vi "(SubVI)_2Ddisplay_direct_doppler_Ver6.vi"(0 "Data":dbl[][](array[numeric]), 1 "Image Avg 2D":dbl, 5 "zero array":dbl[][](array[numeric])=array250x513[128250 elements], 7 "first row":dbl[](array[numeric])=[0.0, 0.69647, 1.3934, 2.0908, 2.7886, 3.4868, 4.1855, 4.8847, 5.5842, 6.2843, 6.9848, 7.6857, 8.3871, 9.0889, 9.7912, 10.494, 11.197, 11.901, 12.605, 13.309, 14.014, 14.72, 15.426, 16.132, 16.839, 17.546, 18.254, 18.962, 19.67, 20.379, 21.089, 21.799, 22.509, 23.22, 23.932, 24.643, 25.356, 26.068, 26.781, 27.495, 28.209, 28.924, 29.639, 30.354, 31.07, 31.786, 32.503, 33.221, 33.938, 34.656, 35.375, 36.094, 36.814, 37.534, 38.255, 38.976, 39.697, 40.419, 41.141, 41.864, 42.588, 43.311, 44.036, 44.76, 45.486, 46.211, 46.937, 47.664, 48.391, 49.119, 49.847, 50.575, 51.304, 52.034, 52.763, 53.494, 54.225, 54.956, 55.688, 56.42, 57.153, 57.886, 58.62, 59.354, 60.089, 60.824, 61.559, 62.295, 63.032, 63.769, 64.506, 65.244, 65.983, 66.722, 67.461, 68.201, 68.942, 69.683, 70.424, 71.166, 71.908, 72.651, 73.394, 74.138, 74.882, 75.627, 76.372, 77.118, 77.864, 78.611, 79.358, 80.106, 80.854, 81.602, 82.352, 83.101, 83.851, 84.602, 85.353, 86.104, 86.857, 87.609, 88.362, 89.116, 89.87, 90.624, 91.379, 92.135, 92.891, 93.647, 94.404, 95.162, 95.92, 96.678, 97.437, 98.197, 98.957, 99.717, 100.48, 101.24, 102.0, 102.76, 103.53, 104.29, 105.05, 105.82, 106.58, 107.35, 108.12, 108.88, 109.65, 110.42, 111.18, 111.95, 112.72, 113.49, 114.26, 115.03, 115.8, 116.57, 117.35, 118.12, 118.89, 119.67, 120.44, 121.21, 121.99, 122.77, 123.54, 124.32, 125.1, 125.87, 126.65, 127.43, 128.21, 128.99, 129.77, 130.55, 131.33, 132.11, 132.9, 133.68, 134.46, 135.25, 136.03, 136.81, 137.6, 138.39, 139.17, 139.96, 140.75, 141.53, 142.32, 143.11, 143.9, 144.69, 145.48, 146.27, 147.07, 147.86, 148.65, 149.44, 150.24, 151.03, 151.83, 152.62, 153.42, 154.21, 155.01, 155.81, 156.61, 157.41, 158.2, 159.0, 159.8, 160.61, 161.41, 162.21, 163.01, 163.81, 164.62, 165.42, 166.22, 167.03, 167.84, 168.64, 169.45, 170.26, 171.06, 171.87, 172.68, 173.49, 174.3, 175.11, 175.92, 176.73, 177.54, 178.36, 179.17, 179.98, 180.8, 181.61, 182.43, 183.24, 184.06, 184.88, 185.69, 186.51, 187.33, 188.15, 188.97, 189.79, 190.61, 191.43, 192.25, 193.07, 193.9, 194.72, 195.54, 196.37, 197.19, 198.02, 198.85, 199.67, 200.5, 201.33, 202.16, 202.99, 203.82, 204.65, 205.48, 206.31, 207.14, 207.97, 208.8, 209.64, 210.47, 211.31, 212.14, 212.98, 213.81, 214.65, 215.49, 216.33, 217.16, 218.0, 218.84, 219.68, 220.52, 221.37, 222.21, 223.05, 223.89, 224.74, 225.58, 226.43, 227.27, 228.12, 228.96, 229.81, 230.66, 231.51, 232.36, 233.2, 234.05, 234.9, 235.76, 236.61, 237.46, 238.31, 239.17, 240.02, 240.87, 241.73, 242.59, 243.44, 244.3, 245.16, 246.01, 246.87, 247.73, 248.59, 249.45, 250.31, 251.17, 252.04, 252.9, 253.76, 254.63, 255.49, 256.36, 257.22, 258.09, 258.95, 259.82, 260.69, 261.56, 262.43, 263.3, 264.17, 265.04, 265.91, 266.78, 267.66, 268.53, 269.4, 270.28, 271.15, 272.03, 272.9, 273.78, 274.66, 275.54, 276.42, 277.29, 278.17, 279.05, 279.94, 280.82, 281.7, 282.58, 283.47, 284.35, 285.24, 286.12, 287.01, 287.89, 288.78, 289.67, 290.56, 291.45, 292.33, 293.22, 294.12, 295.01, 295.9, 296.79, 297.68, 298.58, 299.47, 300.37, 301.26, 302.16, 303.06, 303.95, 304.85, 305.75, 306.65, 307.55, 308.45, 309.35, 310.25, 311.16, 312.06, 312.96, 313.87, 314.77, 315.68, 316.58, 317.49, 318.4, 319.31, 320.22, 321.12, 322.03, 322.95, 323.86, 324.77, 325.68, 326.59, 327.51, 328.42, 329.34, 330.25, 331.17, 332.09, 333.0, 333.92, 334.84, 335.76, 336.68, 337.6, 338.52, 339.44, 340.37, 341.29, 342.21, 343.14, 344.06, 344.99, 345.91, 346.84, 347.77, 348.7, 349.63, 350.56, 351.49, 352.42, 353.35, 354.28, 355.21, 356.15, 357.08, 358.02, 358.95, 359.89, 360.82, 361.76, 362.7, 363.64, 364.58, 365.52, 366.46, 367.4, 368.34, 369.28, 370.23, 371.17, 372.11, 373.06, 374.01, 374.95, 375.9, 376.85, 377.79, 378.74, 379.69, 380.64, 381.6, 382.55, 383.5, 384.45, 385.41, 386.36, 387.32, 388.27, 389.23, 390.18, 391.14, 392.1, 393.06, 394.02, 394.98, 395.94, 396.9, 397.86, 398.83, 399.79, 400.76, 401.72, 402.69, 403.65, 404.62, 405.59, 406.56, 407.53, 408.5, 409.47, 410.44, 411.41, 412.38, 413.35, 414.33, 415.3, 416.28, 417.25, 418.23, 419.21, 420.19, 421.16, 422.14, 423.12, 424.1, 425.09, 426.07, 427.05, 428.03, 429.02, 430.0, 430.99, 431.97, 432.96, 433.95, 434.94, 435.93, 436.91, 437.91, 438.9, 439.89, 440.88, 441.87, 442.87, 443.86, 444.86, 445.85, 446.85, 447.85, 448.84, 449.84, 450.84, 451.84, 452.84, 453.84, 454.85, 455.85, 456.85, 457.86, 458.86, 459.87, 460.87, 461.88, 462.89, 463.9, 464.91, 465.92, 466.93, 467.94, 468.95, 469.96, 470.98, 471.99, 473.01, 474.02, 475.04, 476.05, 477.07, 478.09, 479.11, 480.13, 481.15, 482.17, 483.19, 484.22, 485.24, 486.26, 487.29, 488.31, 489.34, 490.37, 491.4, 492.42, 493.45, 494.48, 495.51, 496.55, 497.58, 498.61, 499.64, 500.68, 501.71, 502.75, 503.79, 504.82, 505.86, 506.9, 507.94, 508.98, 510.02, 511.06, 512.1, 513.15, 514.19, 515.24, 516.28, 517.33, 518.37, 519.42, 520.47, 521.52, 522.57, 523.62, 524.67, 525.72, 526.77, 527.83, 528.88, 529.94, 530.99, 532.05, 533.1, 534.16, 535.22, 536.28, 537.34, 538.4, 539.46, 540.53, 541.59, 542.65, 543.72, 544.78, 545.85, 546.91, 547.98, 549.05, 550.12, 551.19, 552.26, 553.33, 554.4, 555.48, 556.55, 557.62, 558.7, 559.77, 560.85, 561.93, 563.01, 564.09, 565.17, 566.25, 567.33, 568.41, 569.49, 570.57, 571.66, 572.74, 573.83, 574.92, 576.0, 577.09, 578.18, 579.27, 580.36, 581.45, 582.54, 583.63, 584.73, 585.82, 586.92, 588.01, 589.11, 590.21, 591.3, 592.4, 593.5, 594.6, 595.7, 596.8, 597.91, 599.01, 600.11, 601.22, 602.33, 603.43, 604.54, 605.65, 606.76, 607.87, 608.98, 610.09, 611.2, 612.31, 613.42, 614.54, 615.65, 616.77, 617.89, 619.0, 620.12, 621.24, 622.36, 623.48, 624.6, 625.72, 626.85, 627.97, 629.09, 630.22, 631.34, 632.47, 633.6, 634.73, 635.86, 636.99, 638.12, 639.25, 640.38, 641.51, 642.65, 643.78, 644.92, 646.05, 647.19, 648.33, 649.47, 650.6, 651.74, 652.89, 654.03, 655.17, 656.31, 657.46, 658.6, 659.75, 660.89, 662.04, 663.19, 664.34, 665.49, 666.64, 667.79, 668.94, 670.09, 671.25, 672.4, 673.55, 674.71, 675.87, 677.02, 678.18, 679.34, 680.5, 681.66, 682.82, 683.99, 685.15, 686.31, 687.48, 688.64, 689.81, 690.98, 692.14, 693.31, 694.48, 695.65, 696.82, 697.99, 699.17, 700.34, 701.52, 702.69, 703.87, 705.04, 706.22, 707.4, 708.58, 709.76, 710.94, 712.12, 713.3, 714.48, 715.67, 716.85, 718.04, 719.22, 720.41, 721.6, 722.79, 723.98, 725.17, 726.36, 727.55, 728.74, 729.93, 731.13, 732.32, 733.52, 734.72, 735.91, 737.11, 738.31, 739.51, 740.71, 741.91, 743.11, 744.32, 745.52, 746.72, 747.93, 749.14, 750.34, 751.55, 752.76, 753.97, 755.18, 756.39, 757.6, 758.81, 760.03, 761.24, 762.46, 763.67, 764.89, 766.1, 767.32, 768.54, 769.76, 770.98, 772.2, 773.42, 774.65, 775.87, 777.1, 778.32, 779.55, 780.77, 782.0, 783.23, 784.46, 785.69, 786.92, 788.15, 789.38, 790.61, 791.85, 793.08, 794.32, 795.55, 796.79, 798.03, 799.27, 800.51, 801.75, 802.99, 804.23, 805.47, 806.72, 807.96, 809.2, 810.45, 811.7, 812.94, 814.19, 815.44, 816.69, 817.94, 819.19, 820.44, 821.69, 822.95, 824.2, 825.46, 826.71, 827.97, 829.23, 830.48, 831.74, 833.0, 834.26, 835.52, 836.78, 838.05, 839.31, 840.57, 841.84, 843.1, 844.37, 845.64, 846.9, 848.17, 849.44, 850.71, 851.98, 853.25, 854.53, 855.8, 857.07, 858.35, 859.62, 860.9, 862.18, 863.45, 864.73, 866.01, 867.29, 868.57, 869.85, 871.13, 872.42, 873.7, 874.98, 876.27, 877.55, 878.84, 880.13, 881.42, 882.7, 883.99, 885.28, 886.57, 887.87, 889.16, 890.45, 891.74, 893.04, 894.33, 895.63, 896.92, 898.22, 899.52, 900.82, 902.12, 903.42, 904.72, 906.02, 907.32, 908.62, 909.93, 911.23, 912.53, 913.84, 915.15, 916.45, 917.76, 919.07, 920.38, 921.69, 923.0, 924.31, 925.62, 926.93, 928.24, 929.56, 930.87, 932.19, 933.5, 934.82, 936.13, 937.45, 938.77, 940.09, 941.41, 942.73, 944.05, 945.37, 946.69, 948.01, 949.34, 950.66, 951.98, 953.31, 954.63, 955.96, 957.29, 958.61, 959.94, 961.27, 962.6, 963.93, 965.26, 966.59, 967.92, 969.26, 970.59, 971.92, 973.26, 974.59, 975.93, 977.26, 978.6, 979.93, 981.27, 982.61, 983.95, 985.29, 986.63, 987.97, 989.31, 990.65, 991.99, 993.33, 994.68, 996.02, 997.36, 998.71, 1000.1, 1001.4, 1002.7, 1004.1, 1005.4, 1006.8, 1008.1, 1009.5, 1010.8, 1012.2, 1013.5, 1014.9, 1016.2, 1017.6, 1018.9, 1020.3, 1021.6, 1023.0], 9 "input cluster 3":T1={"data_points"=250, "camera_pixel"=1024, "zero array"=array250x513[128250 elements], "complex zero array"=array250x1026[256500 elements]}, 11 "ROI":cluster{"ROI_Bot":i32, "ROI_Top":i32}, 12 "VelcityProfile":dbl[][](array[numeric]), 13 "Numeric":dbl=2.5e-05) -> (8 "complex_depth_profile 2":dbl[][](array[numeric]), 10 "velocity_profile":dbl[][](array[numeric]), 15 "error out 4":errorcluster)   [LabVIEW 2019]
uses:
  SD_OCT_Ver4.dll
panel:
  out "buffer out 3":dbl[][](array[numeric])
  in  "error in (no error) 3":errorcluster
  out "Depth_profile":dbl[][](array[numeric])
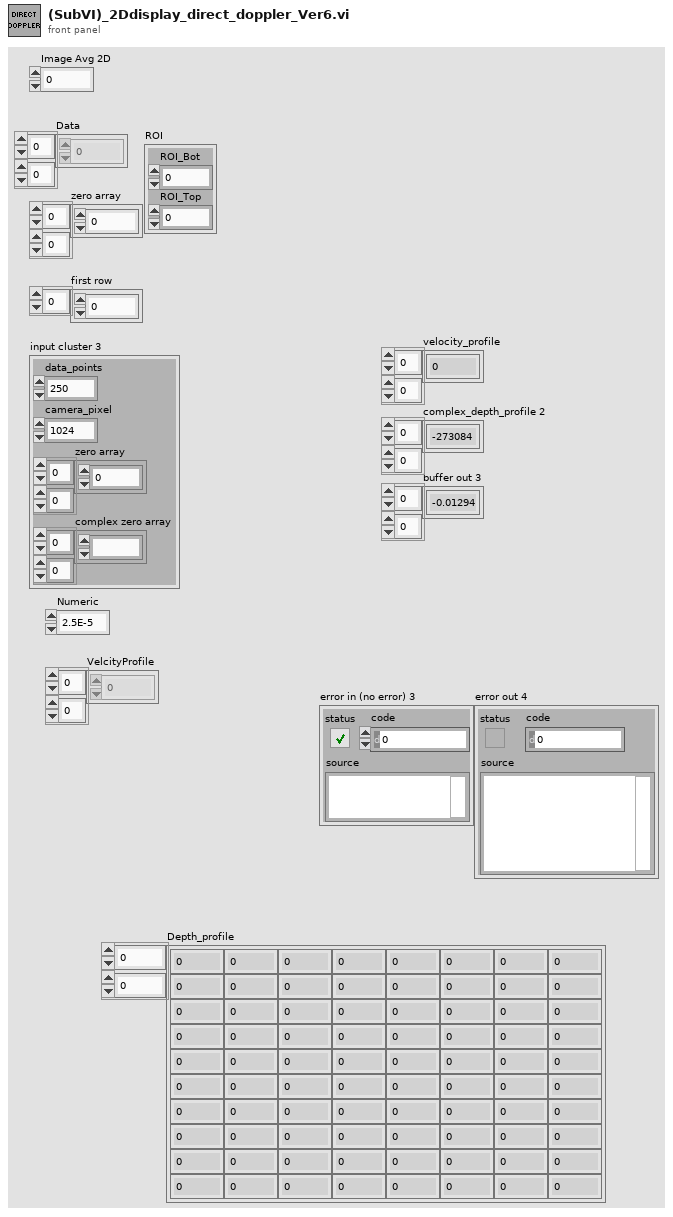
[diagram p1: front panel]
types:
  T1 = cluster{"data_points":i32, "camera_pixel":i32, "zero array":dbl[][], "complex zero array":dbl[][]}
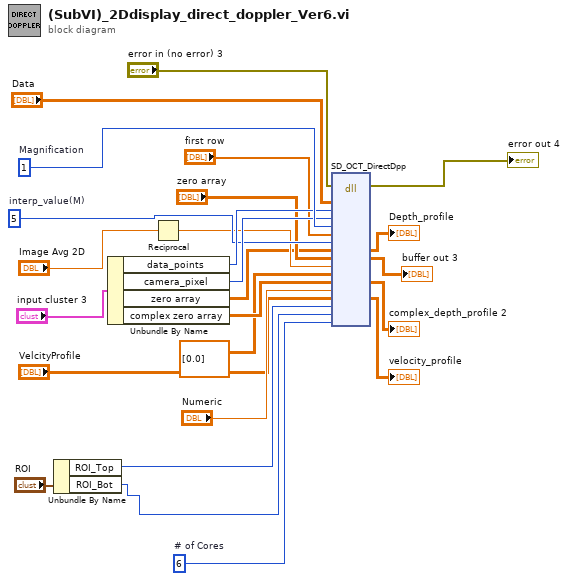
[diagram p0: block diagram]
diagram:
  w12 = 5  # interp_value(M)
  w13 = 6  # # of Cores
  w21 = 1  # Magnification
  n1 = Unbundle By Name("ROI") -> ("ROI_Top"=w2:i32, "ROI_Bot"=w1:i32)
  n2 = Unbundle By Name("input cluster 3") -> ("data_points"=w18:i32, "camera_pixel"=w17:i32, "zero array"=w8:dbl[][], "complex zero array"=w16:dbl[][])
  n3 = Reciprocal(x="Image Avg 2D") -> (1/x=w9:dbl)
  n4 = dll-call lib="C:/Users/hesfandi/Desktop/labview/LabViewCode/SD_OCT_Ver4.dll" fn="SD_OCT_DirectDpp"(error in="error in (no error) 3", "Data"="Data", "data_points"=w18, "camera_pixel"=w17, "Magnification"=w21, "new_index"="first row", "interp_value"=w12, "depth_profile"=w8, "buffer"="zero array", "alpha"=w9, "weight"=dbl[][] [[0.0]] ("complex zero array"), "complex_depth_profile"=w16, "Delta_t"="Numeric", "VelcityProfile"="VelcityProfile", "ROI_Top"=w2, "ROI_Bot"=w1, "core_number"=w13) -> (error out=→"error out 4":errorcluster, "depth_profile"=→"Depth_profile":dbl[][], "buffer"=→"buffer out 3":dbl[][], "complex_depth_profile"=→"complex_depth_profile 2":dbl[][], "VelcityProfile"=→"velocity_profile":dbl[][])  [unwired: 15 in, 1 out]
